vi "Calibration.vi"   [LabVIEW 2012]
uses:
  Global Variables.vi
  Global Refnums.vi
types:
  T1 = enum16{"open", "replace", "create", "open or create", "replace or create", "replace or create with confirmation"}
  T2 = typedef "WPI_AnalogChannelDevRef.ctl" = cluster{"DevStatus":errorcluster, "Analog Module":T3, "Analog Channel":T4}
  T3 = typedef "FPGA_TypedefAnalogModule.ctl" = enum16{"Analog Module 1", "Analog Module 2"}
  T4 = typedef "FPGA_AIChannel.ctl" = enum8{"AI 1", "AI 2", "AI 3", "AI 4", "AI 5", "AI 6", "AI 7", "AI 8", "Invalid"}
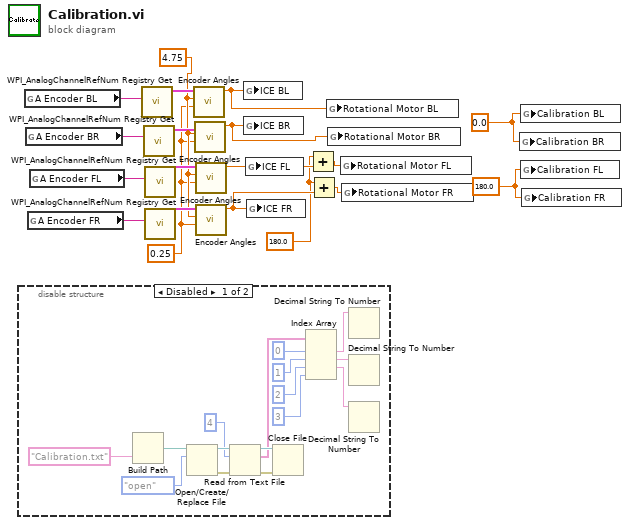
[diagram p0: block diagram]
diagram:
  w1 = 180.0
  w12 = 0.25
  w13 = 4.75
  w18 = 0.0
  w19 = 180.0
  n1 = disable-structure shown="Disabled" {
    frame Disabled {
      n2 = Build Path(name or relative path="Calibration.txt") -> (appended path=w34:path)  [unwired: 1 in]
      n3 = Open/Create/Replace File(file path (use dialog)=w34, operation (0:open)=T1."open") -> (refnum out=w29:refnum<file>, error out=w28:errorcluster)  [unwired: 1 in, 4 out]
      n4 = Read from Text File(file (use dialog)=w29, count=4, error in=w28) -> (refnum out=w32:refnum<file>, text=w30:string[], error out=w31:errorcluster)  [unwired: 2 out]
      n5 = Close File(refnum=w32, error in=w31) -> ()  [unwired: 2 out]
      n6 = Index Array(array=w30, index #1=0 ("index"), index #2=1 ("index"), index #3=2 ("index"), index #4=3 ("index")) -> (element #1=w22:string, element #2=w21:string, element #3=w20:string)  [unwired: 1 out]
      n7 = Decimal String To Number(string=w22) -> ()  [unwired: 1 in, 3 out]
      n8 = Decimal String To Number(string=w21) -> ()  [unwired: 1 in, 3 out]
      n9 = Decimal String To Number(string=w20) -> ()  [unwired: 1 in, 3 out]
    }
    frame Enabled {
    }
  }
  n10 = global read "Global Refnums.vi" "A Encoder BL"() -> (w11:string)
  n11 = global read "Global Refnums.vi" "A Encoder BR"() -> (w10:string)
  n12 = global read "Global Refnums.vi" "A Encoder FR"() -> (w8:string)
  n13 = global read "Global Refnums.vi" "A Encoder FL"() -> (w9:string)
  n14 = call <vilib>:"WPI_AnalogChannelRefNum Registry Get.vi"("refnum name"=w11) -> ("AIDeviceRef"=w17:T2)  [unwired: 9 in, 1 out]
  n15 = call <vilib>:"WPI_AnalogChannelRefNum Registry Get.vi"("refnum name"=w10) -> ("AIDeviceRef"=w16:T2)  [unwired: 9 in, 1 out]
  n16 = call <vilib>:"WPI_AnalogChannelRefNum Registry Get.vi"("refnum name"=w9) -> ("AIDeviceRef"=w15:T2)  [unwired: 9 in, 1 out]
  n17 = call <vilib>:"WPI_AnalogChannelRefNum Registry Get.vi"("refnum name"=w8) -> ("AIDeviceRef"=w14:T2)  [unwired: 9 in, 1 out]
  n18 = call "Encoder Angles.vi"("Bottom Voltage"=w12, "Top Voltage"=w13, "AIDeviceRef Encoder"=w17) -> ("Encoder Angle"=w6:dbl)  [unwired: 8 in]
  n19 = call "Encoder Angles.vi"("Bottom Voltage"=w12, "Top Voltage"=w13, "AIDeviceRef Encoder"=w16) -> ("Encoder Angle"=w5:dbl)  [unwired: 8 in]
  n20 = call "Encoder Angles.vi"("Bottom Voltage"=w12, "Top Voltage"=w13, "AIDeviceRef Encoder"=w15) -> ("Encoder Angle"=w7:dbl)  [unwired: 8 in]
  n21 = call "Encoder Angles.vi"("Bottom Voltage"=w12, "Top Voltage"=w13, "AIDeviceRef Encoder"=w14) -> ("Encoder Angle"=w4:dbl)  [unwired: 8 in]
  n22 = global write "Global Variables.vi" "ICE BL"(w6) -> ()
  n23 = global write "Global Variables.vi" "ICE BR"(w5) -> ()
  n24 = global write "Global Variables.vi" "ICE FL"(w7) -> ()
  n25 = global write "Global Variables.vi" "ICE FR"(w4) -> ()
  n26 = Add(x=w1, y=w7) -> (x+y=w3:dbl)
  n27 = Add(x=w1, y=w4) -> (x+y=w2:dbl)
  n28 = global write "Global Variables.vi" "Rotational Motor BL"(w6) -> ()
  n29 = global write "Global Variables.vi" "Rotational Motor BR"(w5) -> ()
  n30 = global write "Global Variables.vi" "Rotational Motor FL"(w3) -> ()
  n31 = global write "Global Variables.vi" "Rotational Motor FR"(w2) -> ()
  n32 = global write "Global Variables.vi" "Calibration BR"(w18) -> ()
  n33 = global write "Global Variables.vi" "Calibration BL"(w18) -> ()
  n34 = global write "Global Variables.vi" "Calibration FL"(w19) -> ()
  n35 = global write "Global Variables.vi" "Calibration FR"(w19) -> ()
